vi "Import Matrix.vi"(10 "PinPositions In":dbl[][](array[numeric])=[[1.0, 0.0, 0.0, 0.0, 0.0, 0.0], [0.0, 1.0, 0.0, 0.0, 0.0, 0.0], [0.0, 0.0, 1.0, 0.0, 0.0, 0.0], [0.0, 0.0, 0.0, 1.0, 0.0, 0.0], [0.0, 0.0, 0.0, 0.0, 1.0, 0.0], [0.0, 0.0, 0.0, 0.0, 0.0, 1.0]]) -> (2 "PinPositions Out":dbl[][](array[numeric]), 3 "Canceled":bool)   [LabVIEW 2013]
panel:
  in  "Cancel":bool
  in  "Ok":bool
  in  "Text Block":string="1.0 0.0 0.0 0.0 0.0 0.0\n0.0 1.0 0.0 0.0 0.0 0.0\n0.0 0.0 1.0 0.0 0.0 0.0\n0.0 0.0 0.0 1.0 0.0 0.0\n0.0 0.0 0.0 0.0 1.0 0.0\n0.0 0.0 0.0 0.0 0.0 1.0"
  # "Paste space and linefeed delimited matrix and press OK"
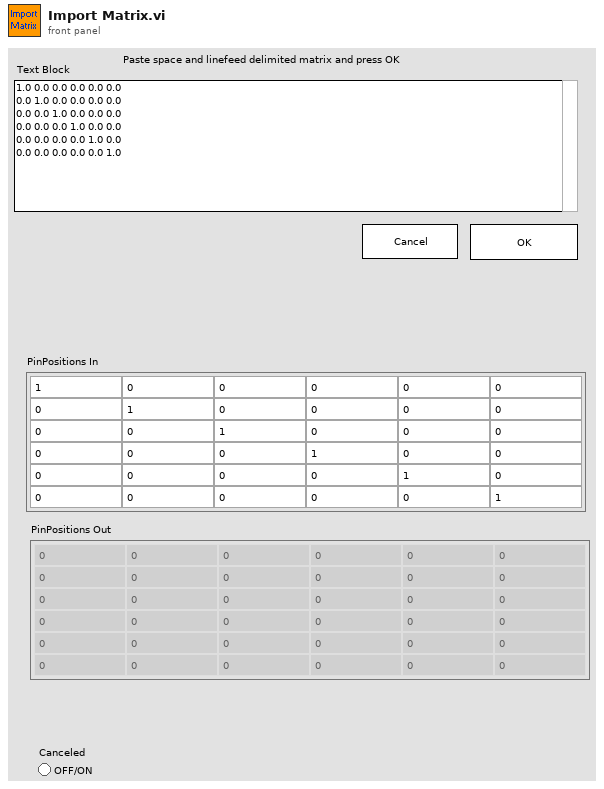
[diagram p1: front panel]
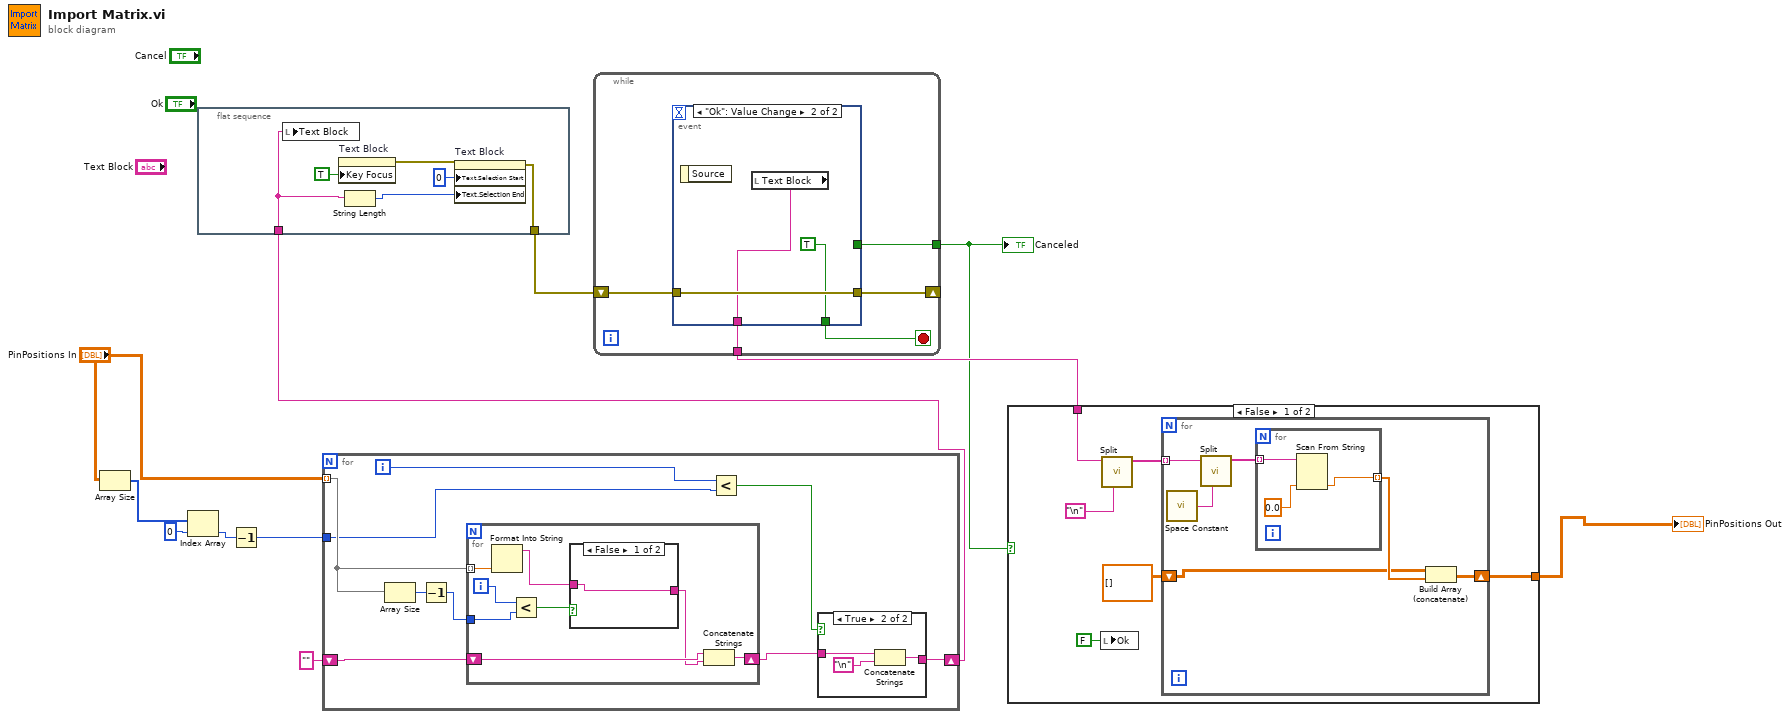
[diagram p0: block diagram]
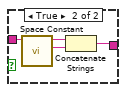
[diagram p3: hidden frame]
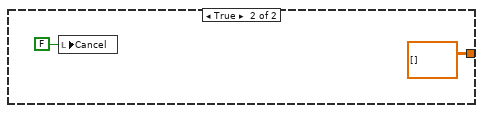
[diagram p4: hidden frame]
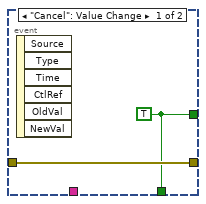
[diagram p5: hidden frame]
diagram:
  n1 = Array Size(array="PinPositions In") -> (size(s)=w8:i32[])
  n2 = Index Array(array=w8, index=0) -> (element=w6:i32)
  n3 = flat-sequence {
    tunnel: [w16] -> w11
    tunnel: w4 -> [w12]
    frame #0 {
      n4 = local write "Text Block"(w12) -> ()
      n5 = property on="Text Block" class="Str"("Key Focus"=TRUE) -> (error out=w14:errorcluster)  [unwired: 2 in, 1 out]
      n6 = String Length(string=w12) -> (length=w13:i32)
      n7 = property on="Text Block" class="Str"(error in=w14, "Text.Selection Start"=u32 0 ("Text.Selection:Start"), "Text.Selection End"=w13) -> (error out=w16:errorcluster)  [unwired: 1 in, 1 out]
    }
  }
  n8 = Decrement(x=w6) -> (x-1=w5:i32)
  n9 = for {
    tunnel: "PinPositions In" -> [w25] mode=indexing
    shift-right: [w18] -> w4
    shift-left: "" -> [w26]
    tunnel: w5 -> [w20]
    i -> [w21]
    n10 = Array Size(array=w25) -> (size(s)=w24:i32)
    n11 = Decrement(x=w24) -> (x-1=w23:i32)
    n12 = for {
      shift-right: [w35] -> w22
      shift-left: w26 -> [w34]
      tunnel: w25 -> [w38] mode=indexing
      tunnel: w23 -> [w31]
      i -> [w32]
      n13 = Format Into String(w38) -> (resulting string=w36:string)  [unwired: 3 in, 1 out]
      n14 = Less?(x=w32, y=w31) -> (x < y?=w37:bool)
      n15 = case shown="False" w37 {
        tunnel: w36 -> [w39 w42]
        tunnel: [w39 w40] -> w33
        frame False {
        }
        frame True {
          n16 = call <vilib>:"Space Constant.vi"() -> ("String"=w41:string)
          n17 = Concatenate Strings(w42, w41) -> (w40:string)
        }
      }
      n18 = Concatenate Strings(w34, w33) -> (w35:string)
    }
    n19 = Less?(x=w21, y=w20) -> (x < y?=w19:bool)
    n20 = case shown="True" w19 {
      tunnel: w22 -> [w27 w30]
      tunnel: [w27 w28] -> w18
      frame False {
      }
      frame True {
        n21 = Concatenate Strings(w30, "\n") -> (w28:string)
      }
    }
  }
  n22 = while {
    shift-right: [w46] -> _
    shift-left: w11 -> [w47]
    tunnel: [w45] -> w9
    tunnel: [w43] -> w10
    stop <- w44 stop-if-true
    n23 = event shown="[1] \"Ok\": Value Change" {
      selector: _ -> [_ _]
      dyn-events: _ -> [_ _]
      timeout: _ -> [_ _]
      tunnel: w47 -> [w49 w52]
      tunnel: [w49 w52] -> w46
      tunnel: [w48 _] -> w45
      tunnel: [w48 TRUE] -> w44
      tunnel: [_ w50] -> w43
      event "Cancel": Value Change {
        w48 = TRUE
        n24 = event-data() -> ()  [unwired: 1 in, 6 out]
      }
      event "Ok": Value Change {
        n25 = event-data() -> ()  [unwired: 1 in, 1 out]
        n26 = local read "Text Block"() -> (w50:string)
      }
    }
  }
  "Canceled" <- w9
  n27 = case shown="False" w9 {
    tunnel: w10 -> [w58 _]
    tunnel: [w55 dbl[][] []] -> w1
    frame False {
      n28 = local write "Ok"(FALSE ("Ok")) -> ()
      n29 = call "Split.vi"("delimiter"="\n", "String"=w58) -> ("Array Result"=w56:string[])  [unwired: 9 in]
      n30 = for {
        tunnel: w56 -> [w64] mode=indexing
        shift-right: [w60] -> w55
        shift-left: dbl[][] [] -> [w59]
        n31 = call <vilib>:"Space Constant.vi"() -> ("String"=w63:string)
        n32 = call "Split.vi"("delimiter"=w63, "String"=w64) -> ("Array Result"=w62:string[])  [unwired: 9 in]
        n33 = for {
          tunnel: w62 -> [w67] mode=indexing
          tunnel: [w65] -> w61 mode=indexing
          n34 = Scan From String(input string=w67, default 1=0.0) -> (output 1=w65:dbl)  [unwired: 3 in, 3 out]
        }
        n35 = Build Array (concatenate)(w59, w61) -> (w60:dbl[][])
      }
    }
    frame True {
      n36 = local write "Cancel"(FALSE ("Cancel")) -> ()
    }
  }
  "PinPositions Out" <- w1
